vi "set_power_level.vi"(8 "error in (no error)":errorcluster, 9 "Power (%)":sgl format="%#_13g", 10 "Layer":u8, 11 "VISA resource name":refnum<visa-resource-name>) -> (0 "error out":errorcluster, 3 "VISA resource name out":refnum<visa-resource-name>)   [LabVIEW 2018]
doc: "Start the active process or continue a process that is in the STOP state."
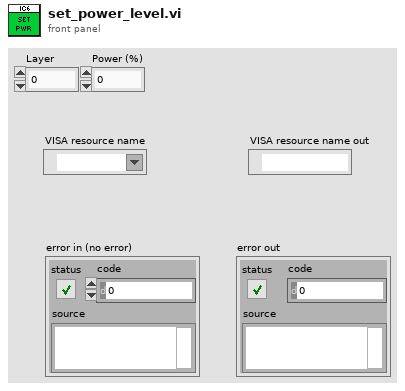
[diagram p1: front panel]
types:
  T1 = enum16{"Source", "General", "Input name", "Process name", "Logic", "Material", "Material name", "Output name", "Process", "Sensor", "Output type", "User message", "Layer", ""}
  T2 = enum16{"Hello", "Query", "Remote action", "Status", "Update"}
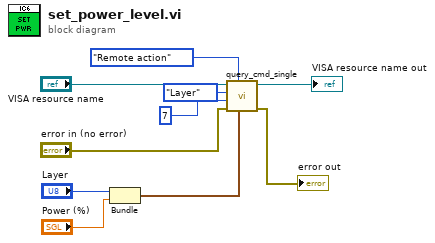
[diagram p0: block diagram]
diagram:
  n1 = Bundle("Layer"="Layer", "Power (%)"="Power (%)") -> (w1:cluster{"Layer":u8, "Power (%)":sgl})  [unwired: 1 in]
  n2 = call "query_cmd_single.vi"("Parameter"=w1, "Command group"=T2."Remote action", "error in (no error)"="error in (no error)", "Command ID"=u8 7, "Command subgroup"=T1."Layer", "VISA resource name"="VISA resource name") -> ("error out"=→"error out":errorcluster, "VISA resource name out"=→"VISA resource name out":refnum<visa-resource-name>)  [unwired: 1 in, 3 out]
